vi "Order_Analysis.vi"(11 "array":waveform(dbl)[](array[waveform])) -> (0 "error out":errorcluster, 3 "order power spectra":T1(array[cluster]) {"order 0" format="%.2p"; "delta order" format="%.2p"; "magnitude" format="%.2f"}, 5 "speed profile":T2 {"speed [RPM]" format="%.2f"; "time [s]" format="%.2f"})   [LabVIEW 2023]
uses:
  <vilib>/addons/Sound and Vibration/Order Analysis/Tach Process/SubVIs/speed profile.ctl
  <vilib>/addons/Sound and Vibration/Order Analysis/Tach Process/OAT Analog Tacho Process (1 Tacho).vi
  <vilib>/addons/Sound and Vibration/Order Analysis/Resample Order Tracking/OAT Convert to Even Angle Signal (N Channels).vi
  <vilib>/addons/Sound and Vibration/Order Analysis/Utility/OAT Output Triggered Even Angle Signal (N Channels).vi
  <vilib>/addons/Sound and Vibration/Order Analysis/Resample Order Tracking/OAT Order Power Spectrum (N Channels).vi
  <vilib>/addons/Sound and Vibration/Order Analysis/Utility/SoundVib_OAUtility.lvlib
  <vilib>/addons/Sound and Vibration/Order Analysis/Tach Process/SoundVib_TachProcess.lvlib
  <vilib>/addons/Sound and Vibration/Order Analysis/Resample Order Tracking/SoundVib_OrderTracking.lvlib
panel:
  out "actual max order":dbl
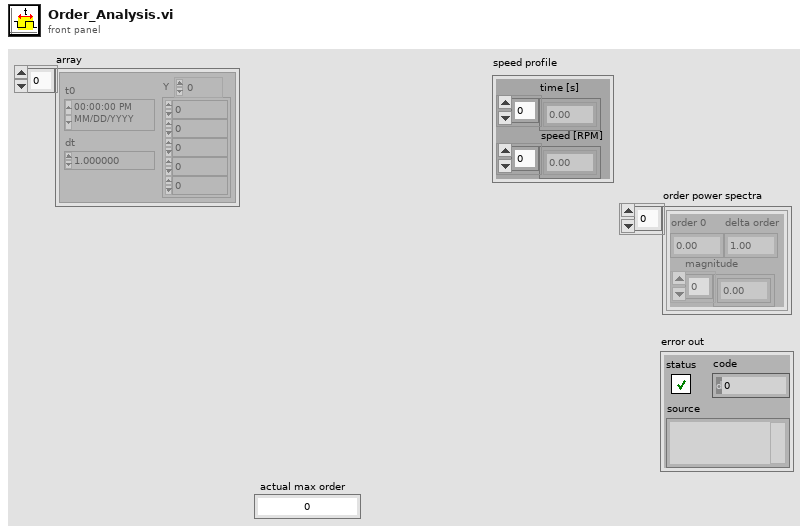
[diagram p1: front panel]
types:
  T1 = cluster{"order 0":dbl, "delta order":dbl, "magnitude":dbl[]}[]
  T2 = typedef "SoundVib_TachProcess.lvlib/speed profile.ctl" = cluster{"time [s]":dbl[], "speed [RPM]":dbl[]}
  T3 = cluster{"averaging mode":enum16{"No averaging", "Vector averaging", "RMS averaging", "Peak hold"}, "weighting mode":enum16{"Linear", "Exponential"}, "number of averages":u32, "linear mode":enum16{"One shot", "Auto restart"}}
  T4 = typedef "svc_Resampled Channel Info.ctl" = cluster{"channel name":string, "description":string, " channel info":T5}
  T5 = typedef "svc_Channel Info.ctl" = cluster{"sensor sensitivity":dbl, "engineering units":T6, "dB reference":dbl, "custom label":string, "weighting filter":T7, "pregain":dbl}
  T6 = typedef "svc_Engineering Units Text Ring.ctl" = u16
  T7 = typedef "svc_Weighting Filter Text Ring.ctl" = u16
  T8 = enum16{"No averaging", "Vector averaging", "RMS averaging", "Peak hold"}
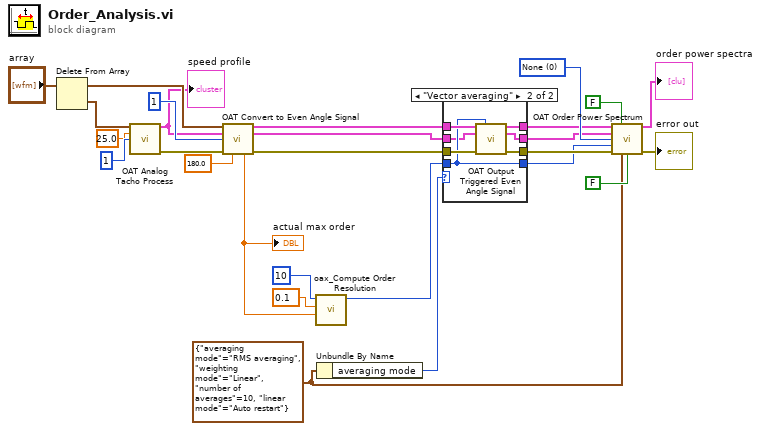
[diagram p0: block diagram]
diagram:
  w24 = T3 {"averaging mode"=enum."RMS averaging", "weighting mode"=enum."Linear", "number of averages"=10, "linear mode"=enum."Auto restart"} ("averaging parameters 2")
  w27 = u32 0 items=["None"=0, "Hanning"=1, "Hamming"=2, "Blackman-Harris"=3, "Exact Blackman"=4, "Blackman"=5, "Flat Top"=6, "4 Term B-Harris"=7, "7 Term B-Harris"=8, "Low Sidelobe"=9, "Gaussian"=62] ("window type")
  n1 = Delete From Array(array="array") -> (deleted portion=w11:waveform(dbl), array with subset deleted=w12:waveform(dbl)[])  [unwired: 2 in]
  n2 = call-poly <vilib>:"OAT Analog Tacho Process.vi"("analog tacho signal"=w11, "threshold (auto)"=25.0, "pulse/revolution (1)"=1) -> ("speed profile"=w7:T2, "error out"=w25:errorcluster)  [unwired: 8 in, 3 out]
  "speed profile" <- w7
  n3 = call-poly <vilib>:"OAT Convert to Even Angle Signal.vi"("scaled signals [EU]"=w12, "speed profile"=w7, "pulse/revolution (1)"=1, "error in (no error)"=w25, "max order (auto)"=180.0) -> ("even-angle signals"=w20:cluster{"r0":dbl, "dr":dbl, "Y":dbl[]}[], "even-angle channel info"=w15:T4[], "actual max order"=w2:dbl, "error out"=w22:errorcluster)  [unwired: 6 in, 1 out]
  "actual max order" <- w2
  n4 = call <vilib>:"oax_Compute Order Resolution.vi"("actual max order"=w2, "order resolution"=0.1 ("order resolution 2"), "block size"=10) -> ("block size out"=w19:i32)  [unwired: 7 in, 1 out]
  n5 = Unbundle By Name(w24) -> ("averaging mode"=w23:T8)
  n6 = case shown="\"Vector averaging\"" w23 {
    tunnel: w22 -> [w31 w38]
    tunnel: [w31 w37] -> w21
    tunnel: w20 -> [w29 w36]
    tunnel: w19 -> [w30 w35]
    tunnel: [w30 w35] -> w18
    tunnel: [w29 w34] -> w17
    tunnel: [w28 w33] -> w16
    tunnel: w15 -> [w28 w32]
    frame "No averaging", Default {
    }
    frame "Vector averaging" {
      n7 = call-poly <vilib>:"OAT Output Triggered Even Angle Signal.vi"("even-angle signals"=w36, "block size"=w35, "even-angle channel info"=w32, "error in (no error)"=w38) -> ("triggered even-angle signals"=w34:cluster{"r0":dbl, "dr":dbl, "Y":dbl[]}[], "even-angle channel info out"=w33:T4[], "error out"=w37:errorcluster)  [unwired: 9 in]
    }
  }
  n8 = call-poly <vilib>:"OAT Order Power Spectrum.vi"("even-angle signals"=w17, "dB on? (T)"=FALSE, "even-angle channel info"=w16, "window"=w27, "block size"=w18, "error in (no error)"=w21, "averaging parameters"=w24, "restart averaging? (F)"=FALSE ("restart averaging (F)")) -> ("order power spectra"=→"order power spectra":T1, "error out"=→"error out":errorcluster)  [unwired: 1 in, 5 out]
